vi "Analog Output - N Channels - Continuous Sampling.vi"() -> ()   [LabVIEW 2019]
uses:
  <vilib>/myRIO/Common/Instrument Driver Framework/myRIO v1.0/UART/vis/myRIO v1.0 Close UART.vi
  <vilib>/myRIO/Instrument Drivers/Onboard IO/AO Continuous/vis/AO Continuous Smart Write.vi
  <vilib>/myRIO/Common/Instrument Driver Framework/Utilities/vis/FPGA Ref Manager.vi
  <vilib>/myRIO/Common/Instrument Driver Framework/ELVIS III v1.0/ELVIS III v1.0 Reset FPGA.vi
  <vilib>/myRIO/Common/Instrument Driver Framework/myRIO v1.0/IRQ/vis/myRIO v1.0 IRQ Info FGV.vi
  <vilib>/myRIO/Common/Instrument Driver Framework/myRIO v1.0/IRQ/vis/myRIO v1.0 Timer IRQ Info FGV.vi
  <vilib>/myRIO/Common/Instrument Driver Framework/myRIO v1.0/IRQ/vis/myRIO v1.0 ISR Agent.vi
  <vilib>/myRIO/Instrument Drivers/Utilities/vis/Reset Index.vi
  <vilib>/myRIO/Common/Instrument Driver Framework/myRIO v1.0/Resource Manager/vis/myRIO v1.0 Block Write Resource Manager.vi
  <vilib>/myRIO/Express VI/Onboard IO/AO/AO Express VI.xnode
  <vilib>/myRIO/Instrument Drivers/Utilities/Utilities.lvlib
  <vilib>/myRIO/Instrument Drivers/Onboard IO/AO Continuous/AO Continuous.lvlib
panel:
  in  "Stop":bool
  in  "AO0 - Sine Amplitude (V)":dbl=5.0 min=-10.0 max=10.0 step=0.1 format="%#_13g"
  in  "AO0 - Sine Frequency (Hz)":dbl=10.0 format="%#_13g"
  in  "AO1 - Triangle Amplitude (V)":dbl=5.0 min=-10.0 max=10.0 step=0.1 format="%#_13g"
  in  "AO1 - Triangle Frequency (Hz)":dbl=10.0 format="%#_13g"
  in  "Generate Waveform":bool
  # "ELVIS III Control IO"
  # "模拟输出N通道"
  # "Overview: Outputs one period of Sine and Triangle waves on Bank A, Channels AO0 and AO1 (A/AO0 and A/AO1).\nInstructions:\n1. Configure the sine wave and triangle wave properties below.\n2. Connect A/AO0 to the positive lead of a load, and connect AGND to the negative lead of the load. Connect A/AO1 to the positive lead of another load, and connect AGND to the negative lead of the corresponding load. AGND is the ground reference terminal for analog output channels.\n3. Run the VI.\n4. Modify the Amplitude and Frequency controls to change the sine and triangle waves.\n5. Press Generate Waveform to output the sine and triangle waves."
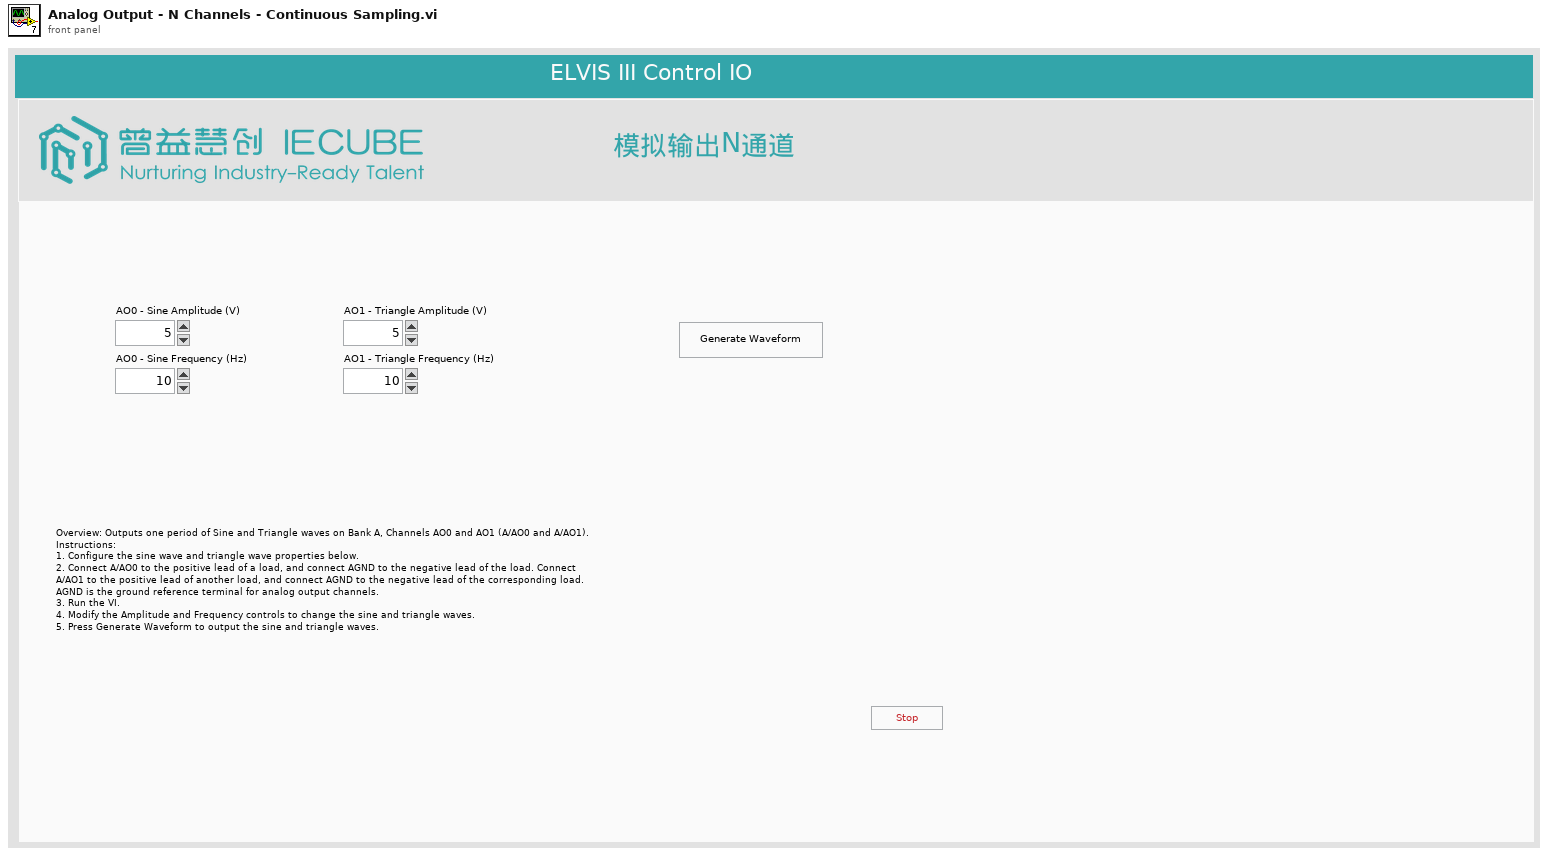
[diagram p1: front panel]
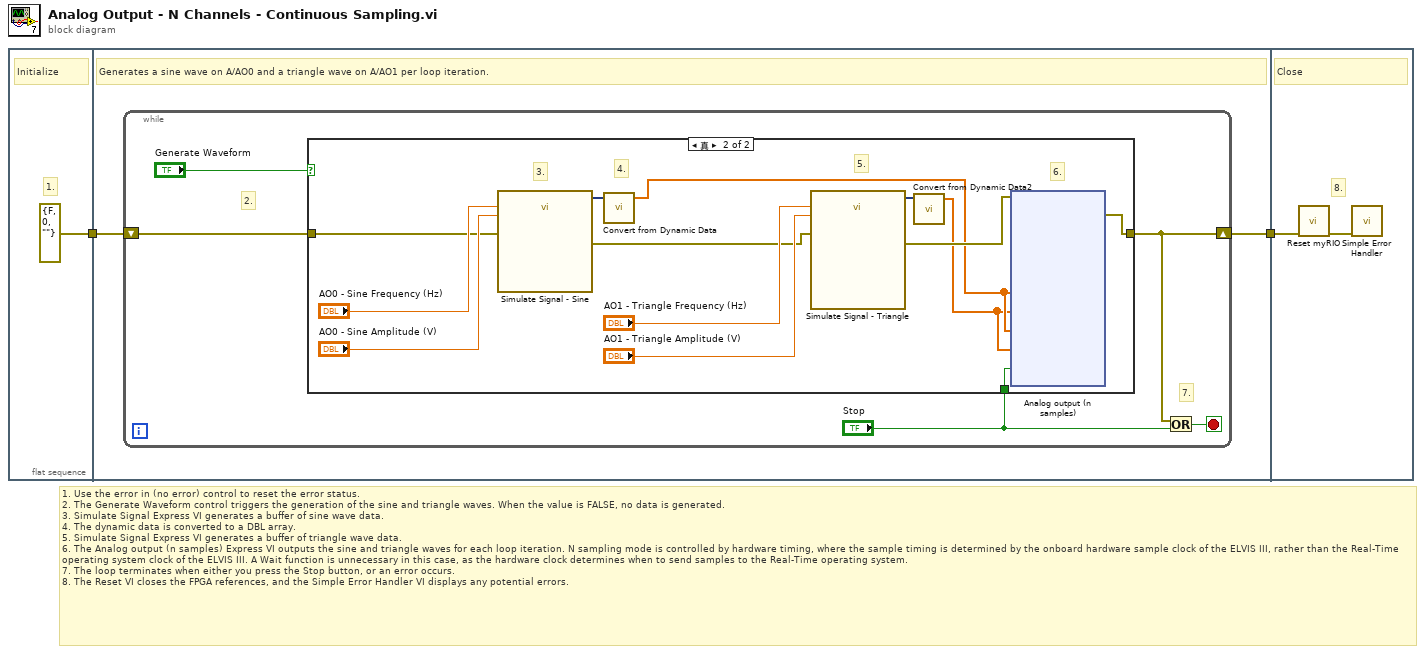
[diagram p0: block diagram]
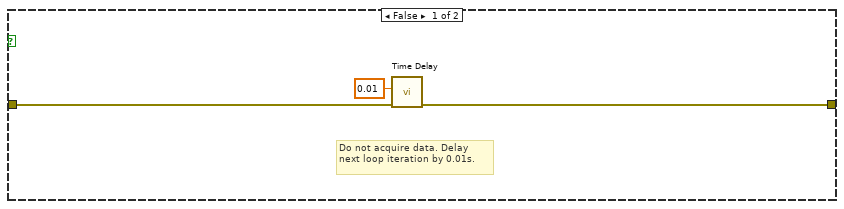
[diagram p2: hidden frame]
diagram:
  # "1. Use the error in (no error) control to reset the error status.\n2. The Generate Waveform control triggers the generation of the sine and triangle waves. When the value is FALSE, no data is generated.\n3. Simulate Signal Express VI generates a buffer of sine wave data.\n4. The dynamic data is converted to a DBL array.\n5. Simulate Signal Express VI generates a buffer of triangle wave data.\n6. The Analog output (n samples) Express VI outputs the sine and triangle waves for each loop iteration. N sampling mode is controlled by hardware timing, where the sample timing is determined by the onboard hardware sample clock of the ELVIS III, rather than the Real-Time operating system clock of the ELVIS III. A Wait function is unnecessary in this case, as the hardware clock determines when to send samples to the Real-Time operating system.\n7. The loop terminates when either you press the Stop button, or an error occurs.\n8. The Reset VI closes the FPGA references, and the Simple Error Handler VI displays any potential errors."
  n1 = flat-sequence {
    tunnel: [errorcluster {"status"=FALSE, "code"=0, "source"=""} ("Error In")] -> w2
    tunnel: [w5] -> w1
    tunnel: w2 -> [w4]
    tunnel: w1 -> [w40]
    frame #0 {
      # "1."
      # "Initialize"
    }
    frame #1 {
      # "Generates a sine wave on A/AO0 and a triangle wave on A/AO1 per loop iteration."
      n2 = while {
        shift-right: [w9] -> w5
        shift-left: w4 -> [w8]
        stop <- w10 stop-if-true
        # "2."
        # "7."
        n3 = case shown="真" "Generate Waveform" {
          tunnel: [w11 w26] -> w9
          tunnel: w8 -> [w12 w22]
          tunnel: "Stop" -> [_ w14]
          frame False {
            # "Do not acquire data. Delay next loop iteration by 0.01s."
            n4 = call "Time Delay"("error in (no error)"=w12, "Delay Time (s)"=0.01) -> ("error out"=w11:errorcluster)  [unwired: 9 in]
          }
          frame True {
            # "6."
            # "5."
            # "4."
            # "3."
            n5 = call "Simulate Signal - Sine"("Frequency"="AO0 - Sine Frequency (Hz)", "Amplitude"="AO0 - Sine Amplitude (V)", "error in (no error)"=w22) -> ("Sine"=w23:dynamicdata, "error out"=w18:errorcluster)  [unwired: 11 in]
            n6 = call "Convert from Dynamic Data"("Dynamic Data Type"=w23) -> ("Array"=w16:dbl[])  [unwired: 3 in]
            n7 = call "Simulate Signal - Triangle"("Frequency"="AO1 - Triangle Frequency (Hz)", "Amplitude"="AO1 - Triangle Amplitude (V)", "error in (no error)"=w18) -> ("Triangle"=w21:dynamicdata, "error out"=w17:errorcluster)  [unwired: 11 in]
            n8 = call "Convert from Dynamic Data2"("Dynamic Data Type"=w21) -> ("Array"=w15:dbl[])  [unwired: 3 in]
            n9 = xnode "Analog output (n samples)"("A/AO0 (Continuous)"=w16, "A/AO1 (Continuous)"=w15, "B/AO0 (Continuous)"=w16, "B/AO1 (Continuous)"=w15, "Stop?"=w14, "error in (no error)"=w17) -> ("error out"=w26:errorcluster)
          }
        }
        n10 = Or(x=w9, y="Stop") -> (x .or. y?=w10:bool)
      }
    }
    frame #2 {
      # "8."
      # "Close"
      n11 = call <vilib>:"Reset myRIO.vi"("error in (no error)"=w40) -> ("error out"=w39:errorcluster)  [unwired: 10 in]
      n12 = call <vilib>:"Simple Error Handler.vi"("error in (no error)"=w39) -> ()  [unwired: 4 in, 5 out]
    }
  }
